vi "ABAPI Dist Create ActiveX Server Name.vi"(1 "name":string) -> (0 "activex name":string)   [LabVIEW 2020]
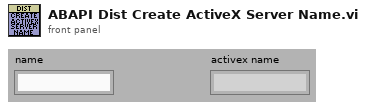
[diagram p1: front panel]
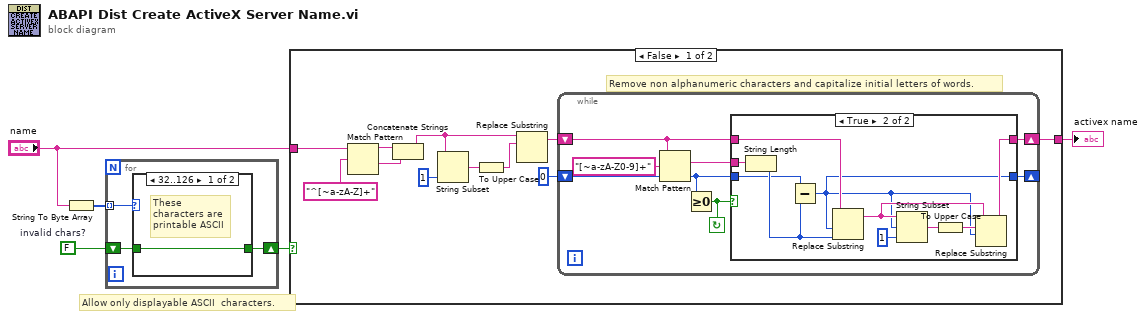
[diagram p0: block diagram]
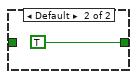
[diagram p4: hidden frame]
diagram:
  w3 = FALSE  # invalid chars?
  # "Allow only displayable ASCII  characters."
  n1 = String To Byte Array(string="name") -> (unsigned byte array=w4:u8[])
  n2 = for {
    tunnel: w4 -> [w8] mode=indexing
    shift-right: [w7] -> w1
    shift-left: w3 -> [w6]
    n3 = case shown="32..126" w8 {
      tunnel: [w9 TRUE ("invalid chars?")] -> w7
      tunnel: w6 -> [w9 _]
      frame 32..126 {
        # "These characters are printable ASCII"
      }
      frame Default {
      }
    }
  }
  n4 = case shown="False" w1 {
    tunnel: [w21 _] -> w5
    tunnel: "name" -> [w11 _]
    frame False {
      # "Remove non alphanumeric characters and capitalize initial letters of words."
      n5 = Match Pattern(string=w11, regular expression="^[~a-zA-Z]+") -> (before substring=w14:string, after substring=w13:string)  [unwired: 3 out]
      n6 = Concatenate Strings(w14, w13) -> (w12:string)
      n7 = String Subset(string=w12, length (rest)=1 ("length (rest)")) -> (substring=w19:string)  [unwired: 1 out]
      n8 = To Upper Case(1:w19) -> (0:w17:string)
      n9 = Replace Substring(4:w17, 5:w12) -> (1:w15:string)  [unwired: 3 out]
      n10 = while {
        shift-left: 0 ("offset past match") -> [w28]
        shift-right: [w23] -> _
        shift-left: w15 -> [w27]
        shift-right: [w26] -> w21
        stop <- w24 continue-if-true
        n11 = Match Pattern(string=w27, regular expression="[~a-zA-Z0-9]+", offset (0)=w28) -> (match substring=w22:string, offset past match=w25:i32)  [unwired: 2 out]
        n12 = Greater Or Equal To 0?(x=w25) -> (x >= 0?=w24:bool)
        n13 = case shown="True" w24 {
          tunnel: w27 -> [w30 w41]
          tunnel: [w30 w37] -> w26
          tunnel: w25 -> [w31 w32]
          tunnel: [w31 w35] -> w23
          tunnel: w22 -> [_ w36]
          frame False {
          }
          frame True {
            n14 = String Length(string=w36) -> (length=w34:i32)
            n15 = Subtract(x=w32, y=w34) -> (x-y=w35:i32)
            n16 = Replace Substring(2:w34, 3:w35, 5:w41) -> (1:w38:string)  [unwired: 2 out]
            n17 = String Subset(string=w38, offset (0)=w35, length (rest)=1 ("length (rest)")) -> (substring=w40:string)
            n18 = To Upper Case(1:w40) -> (0:w39:string)
            n19 = Replace Substring(3:w35, 4:w39, 5:w38) -> (1:w37:string)  [unwired: 2 out]
          }
        }
      }
    }
    frame True {
      # "Return empty if input contains invalid characters."
    }
  }
  "activex name" <- w5
